vi "cRioMain.vi"() -> ()   [LabVIEW 2020]
uses:
  <vilib>/NIScanEngine/faults/Fault.ctl
  Status_cRio.ctl
  Statusword_status.ctl
  ElementDTD.lvlib
panel:
  out "Magnet":bool
  out "Solenoid":bool
  out "Inputs-velocity_actual_value_carrier":i32
  out "Inputs-position_actual_value 2":i32
  out "Inputs-position_actual_value":i32
  out "Verbindung":bool
  out "Ready":bool
  out "TargetReachedY":bool
  out "StatusY":T1
  out "state change":bool
  out "TargetReachedZ":bool
  out "MotorFault":bool
  out "StatusZ":T1
  in  "turnOffM":bool=TRUE
  in  "halt":bool=TRUE
  out "status":T2=enum."1_start_up"
  out "Turn Off":bool
  out "ZielTisch":dbl
  out "Zielhöhe":dbl
  out "fault list":T3[](array[typedef]) caption="Fehlerliste" {"level" items=["Geringfügiger Fehler", "Schwerer Fehler", "Nicht behebbarer Fehler"]}
  out "pcError":bool
  out "Repair":bool
  out "Start":bool
  in  "Stopp":bool
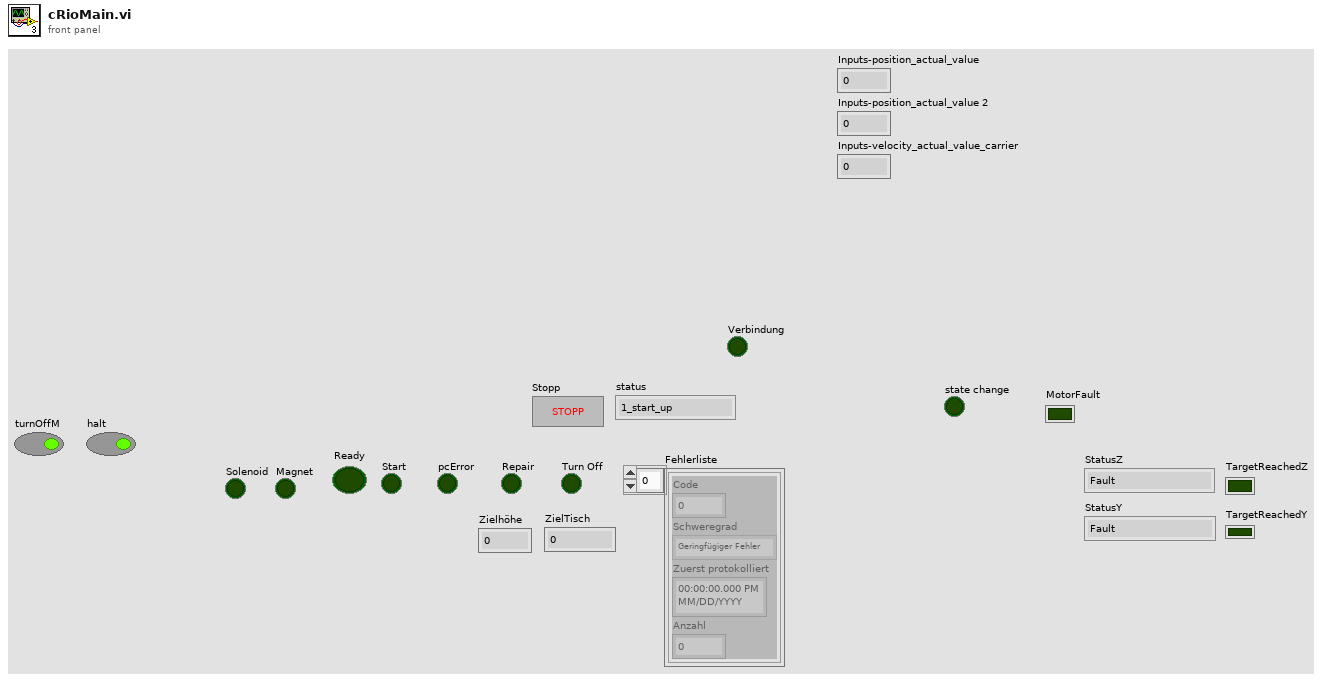
[diagram p1: front panel]
types:
  T1 = typedef "ElementDTD.lvlib/Statusword_status.ctl" = enum16{"Fault", "NOT_READY_TO_SWITCH_ON", "SWITCH_ON_DISABLED", "READY_TO_SWITCH_ON", "SWITCHED_ON", "OPERATION_ENABLE", "QUICK_STOP_ACTIVE"}
  T2 = typedef "ElementDTD.lvlib/Status_cRio.ctl" = enum16{"0_Error", "1_start_up", "4_moving_to_position", "5_measure", "6_DataExport", "7_turnOff"}
  T3 = typedef "Fault.ctl" = cluster{"code":i32, "level":i32, "first reported time":timestamp, "number reported":u32}
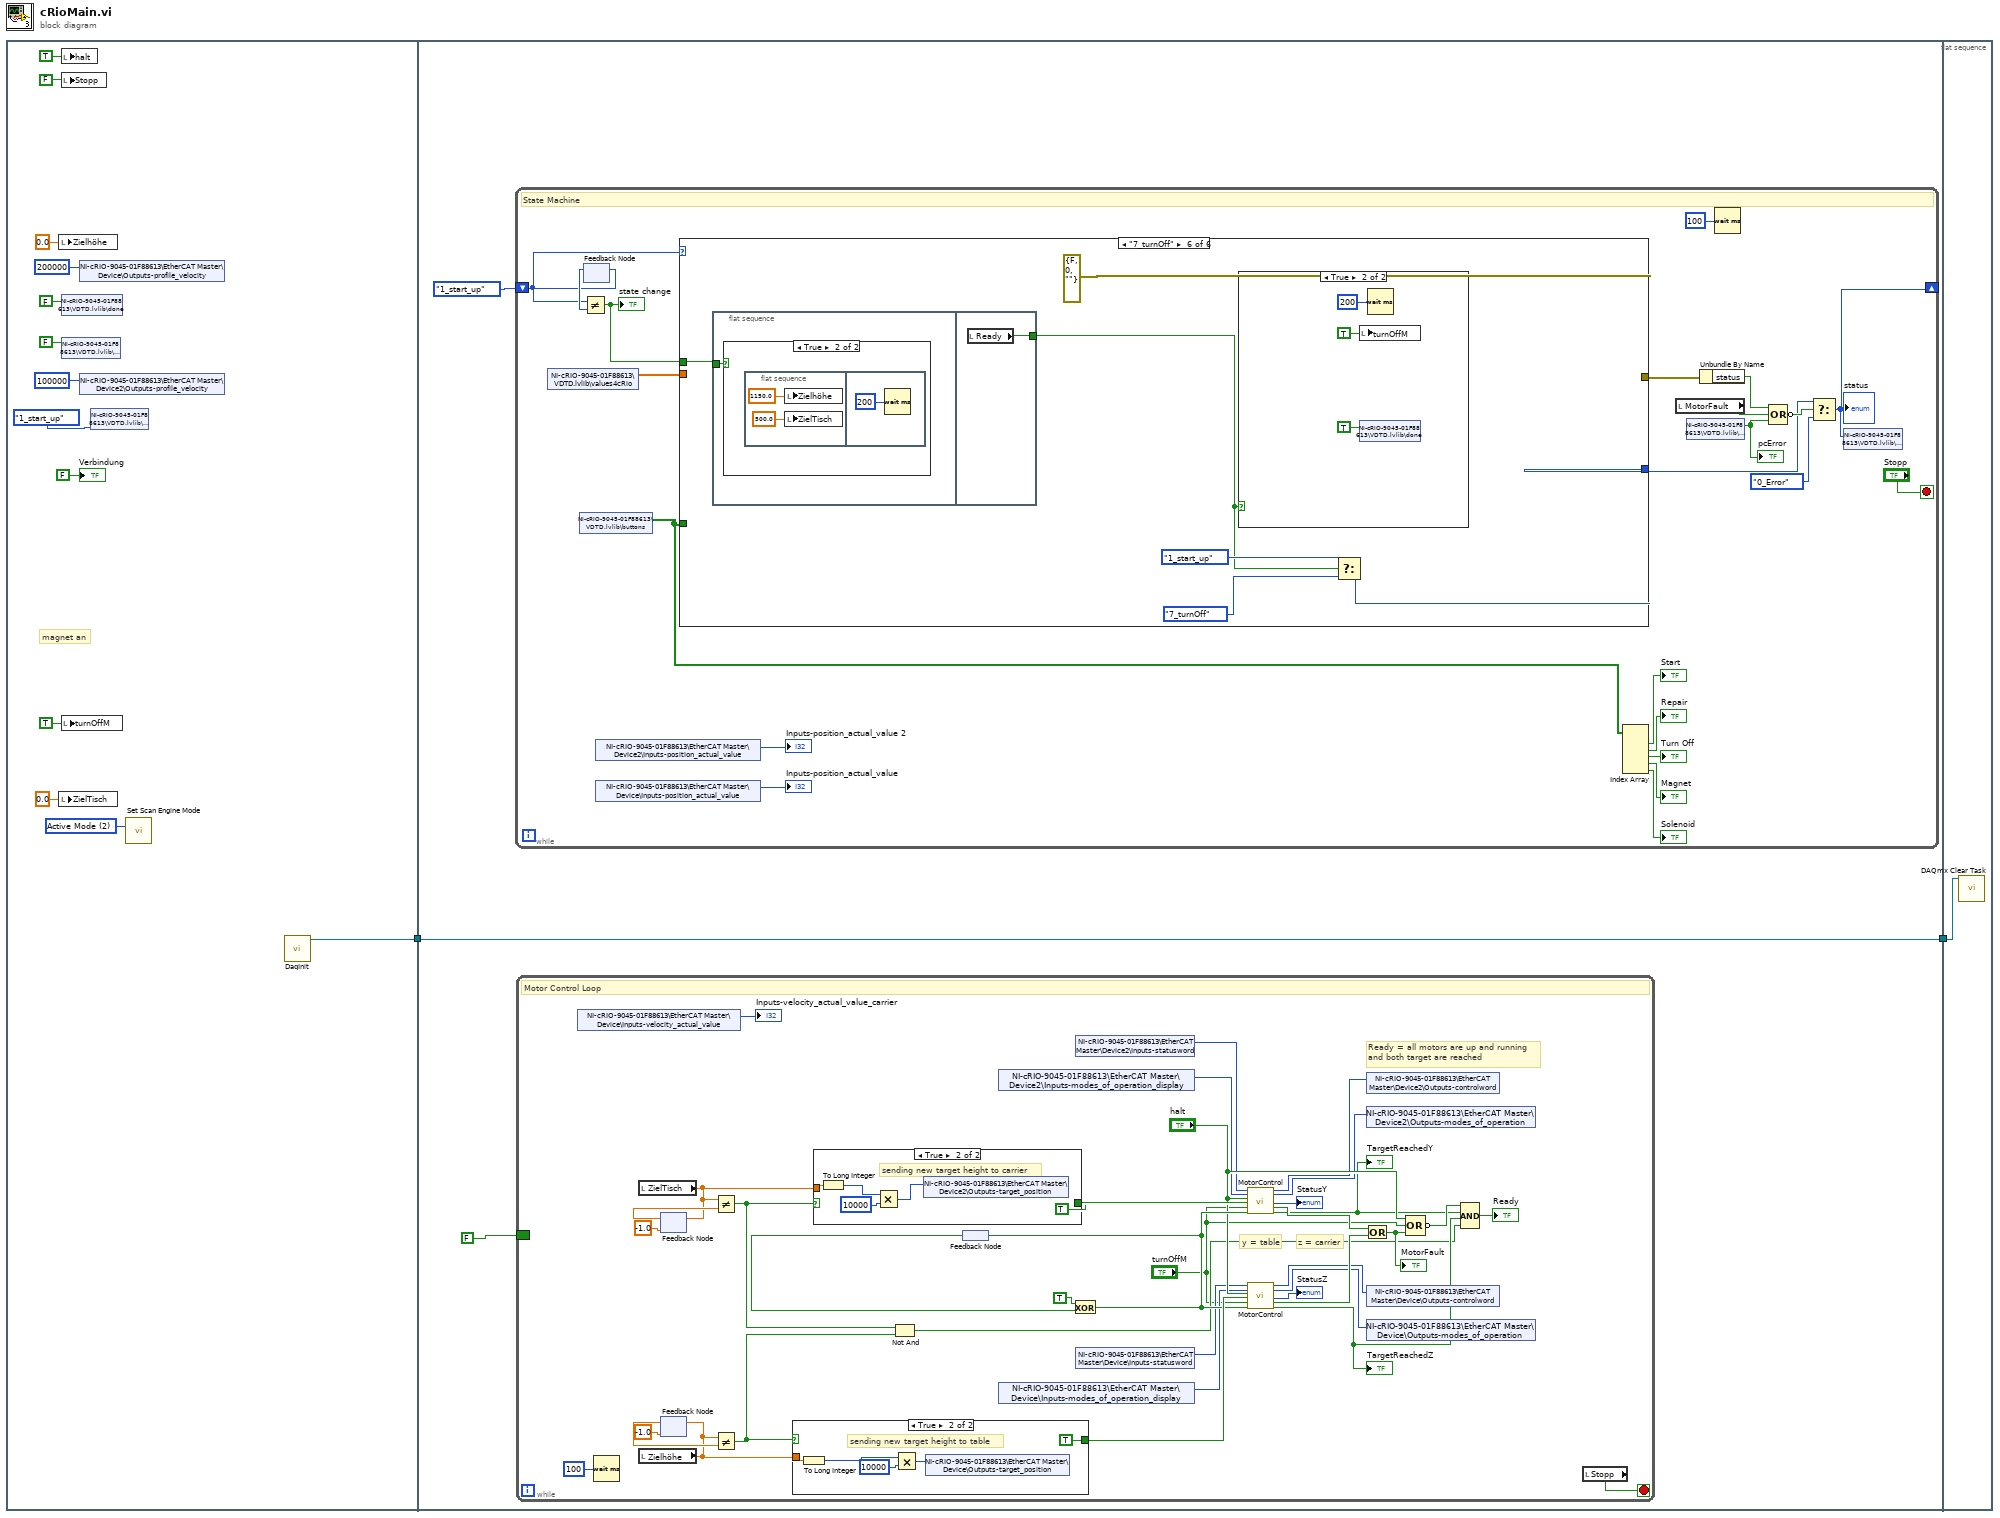
[diagram p0: block diagram]
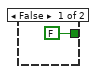
[diagram p2: hidden frame]
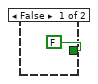
[diagram p3: hidden frame]
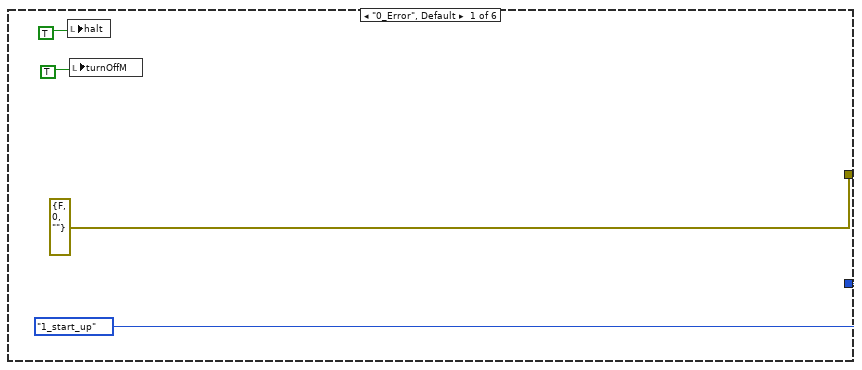
[diagram p4: hidden frame]
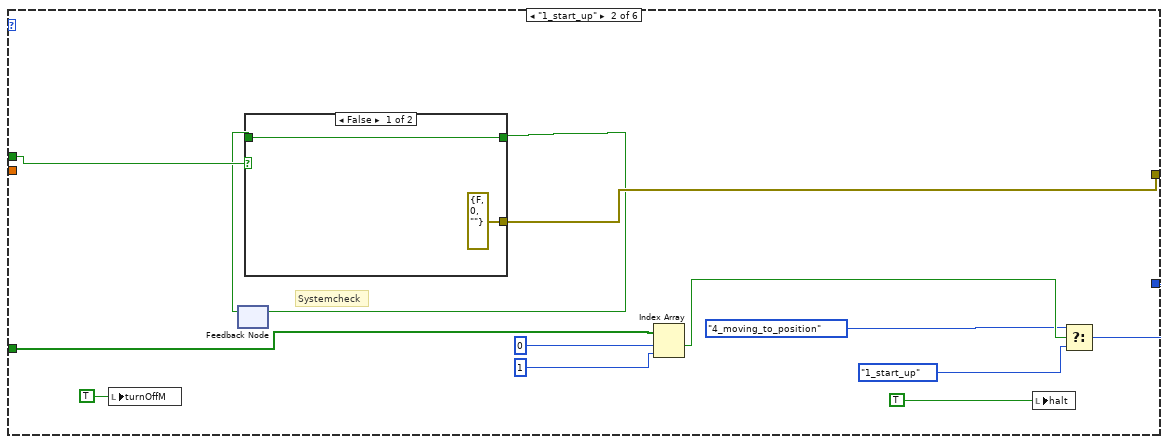
[diagram p5: hidden frame]
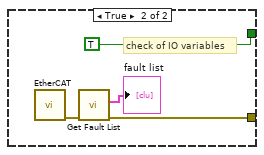
[diagram p6: hidden frame]
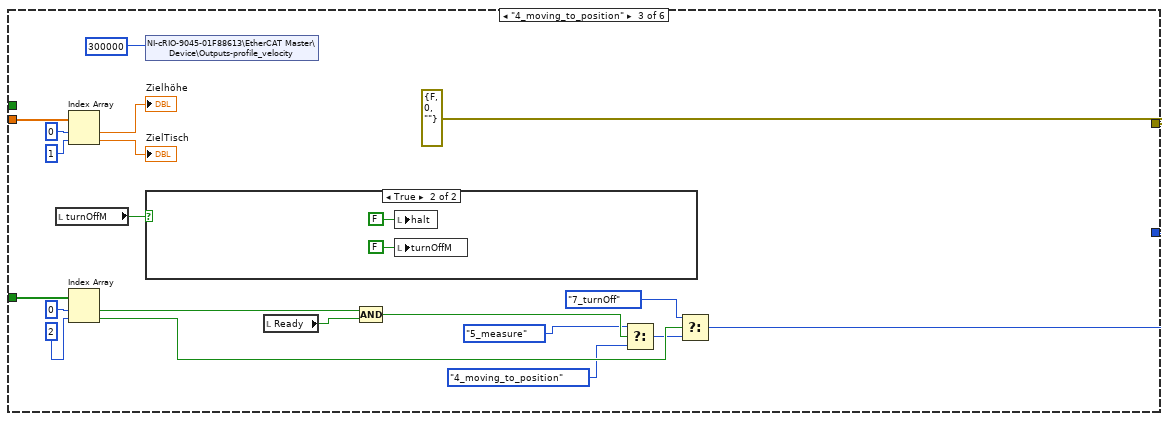
[diagram p7: hidden frame]
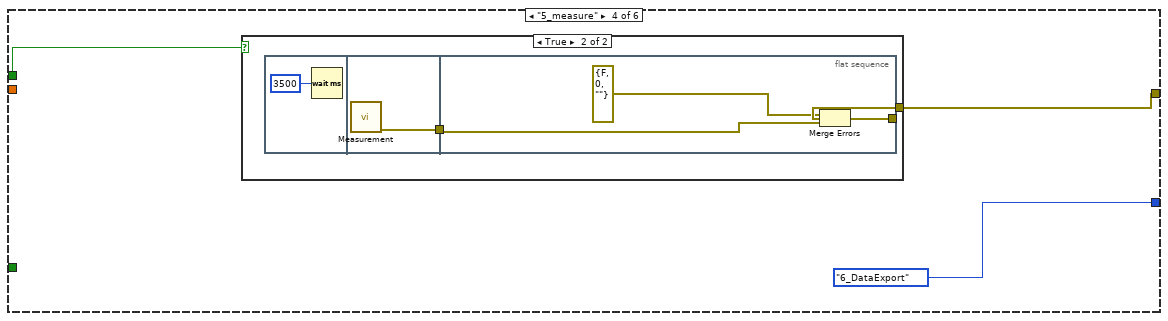
[diagram p9: hidden frame]
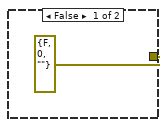
[diagram p10: hidden frame]
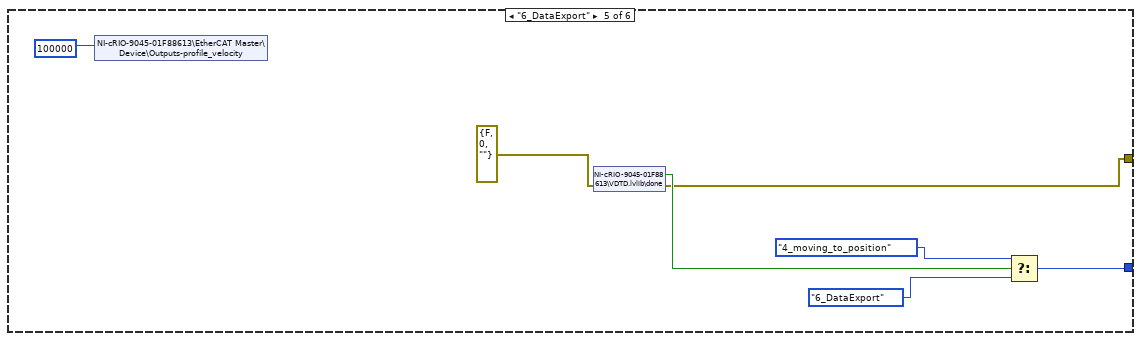
[diagram p11: hidden frame]
diagram:
  n1 = flat-sequence {
    tunnel: [w3] -> w2
    tunnel: w2 -> [w16]
    tunnel: [w16] -> w1
    tunnel: w1 -> [w166]
    frame #0 {
      w6 = 2 items=["Configuration Mode"=1, "Active Mode"=2] ("mode (Active Mode)")
      # "magnet an"
      n2 = local write "Zielhöhe"(0.0 ("Zielhöhe")) -> ()
      n3 = local write "ZielTisch"(0.0 ("ZielTisch")) -> ()
      n4 = local write "halt"(TRUE ("halt")) -> ()
      n5 = local write "Stopp"(FALSE ("Stopp")) -> ()
      n6 = shared-variable "NI-cRIO-9045-01F88613\\VDTD.lvlib\\done"(FALSE ("Done")) -> ()  [unwired: 1 in, 1 out]
      n7 = shared-variable "NI-cRIO-9045-01F88613\\VDTD.lvlib\\error"(FALSE ("Error")) -> ()  [unwired: 1 in, 1 out]
      n8 = local write "turnOffM"(TRUE ("Turn Off")) -> ()
      n9 = shared-variable "NI-cRIO-9045-01F88613\\EtherCAT Master\\Device\\Outputs-profile_velocity"(u32 200000 ("Outputs-profile_velocity")) -> ()  [unwired: 1 in, 1 out]
      n10 = shared-variable "NI-cRIO-9045-01F88613\\EtherCAT Master\\Device2\\Outputs-profile_velocity"(u32 100000 ("Outputs-profile_velocity")) -> ()  [unwired: 1 in, 1 out]
      n11 = shared-variable "NI-cRIO-9045-01F88613\\VDTD.lvlib\\state"(Status_cRio."1_start_up" ("state")) -> ()  [unwired: 1 in, 1 out]
      n12 = call <vilib>:"Set Scan Engine Mode.vi"("mode (Active Mode)"=w6) -> ()  [unwired: 14 in, 1 out]
      n13 = call "DaqInit.vi"() -> ("Refnum out"=w3:refnum<k21>)  [unwired: 10 in, 1 out]
      "Verbindung" <- FALSE ("Verbindung")
    }
    frame #1 {
      n14 = while {
        shift-right: [w73] -> _
        shift-left: Status_cRio."1_start_up" -> [w77]
        stop <- "Stopp" stop-if-true
        # "State Machine"
        n15 = shared-variable "NI-cRIO-9045-01F88613\\VDTD.lvlib\\values4cRio"() -> (w68:dbl[])  [unwired: 1 in, 1 out]
        n16 = shared-variable "NI-cRIO-9045-01F88613\\VDTD.lvlib\\buttons"() -> (w71:bool[])  [unwired: 1 in, 1 out]
        n17 = feedback-in #1(w77) -> ()
        n18 = feedback #1() -> (w80:T2)  [unwired: 1 in]
        n19 = Not Equal?(x=w77, y=w80) -> (x != y?=w72:bool)
        "state change" <- w72
        n20 = shared-variable "NI-cRIO-9045-01F88613\\EtherCAT Master\\Device2\\Inputs-position_actual_value"() -> (→"Inputs-position_actual_value 2":i32)  [unwired: 1 in, 1 out]
        n21 = shared-variable "NI-cRIO-9045-01F88613\\EtherCAT Master\\Device\\Inputs-position_actual_value"() -> (→"Inputs-position_actual_value":i32)  [unwired: 1 in, 1 out]
        n22 = case shown="\"7_turnOff\"" w77 {
          tunnel: [errorcluster {"status"=FALSE, "code"=0, "source"=""} ("error IO") w96 errorcluster {"status"=FALSE, "code"=0, "source"=""} ("error IO") w136 w146 errorcluster {"status"=FALSE, "code"=0, "source"=""} ("error IO")] -> w85
          tunnel: [Status_cRio."1_start_up" w104 w129 Status_cRio."6_DataExport" w145 w154] -> w76
          tunnel: w72 -> [_ w97 _ w135 _ w152]
          tunnel: w71 -> [_ w101 w123 _ _ _]
          tunnel: w68 -> [_ _ w116 _ _ _]
          frame "0_Error", Default {
            n23 = local write "halt"(TRUE ("halt")) -> ()
            n24 = local write "turnOffM"(TRUE ("Turn Off")) -> ()
          }
          frame "1_start_up" {
            # "Systemcheck"
            n25 = local write "turnOffM"(TRUE ("turnOffM")) -> ()
            n26 = feedback #2() -> (w95:bool)  [unwired: 1 in]
            n27 = case shown="False" w97 {
              tunnel: [errorcluster {"status"=FALSE, "code"=0, "source"=""} ("error IO") w110] -> w96
              tunnel: [w106 TRUE ("halt")] -> w94
              tunnel: w95 -> [w106 _]
              frame False {
              }
              frame True {
                # "check of IO variables"
                n28 = call "EtherCAT.vi"() -> ("error IO"=w111:errorcluster)  [unwired: 11 in]
                n29 = call <vilib>:"Get Fault List.vi"("error in (no error)"=w111) -> ("error out"=w110:errorcluster, "fault list"=→"fault list":T3[])  [unwired: 9 in]
              }
            }
            n30 = feedback-in #2(w94) -> ()
            n31 = Index Array(array=w101, index #1=0 ("index"), index #2=1 ("index")) -> (element #1=w100:bool)  [unwired: 1 out]
            n32 = local write "halt"(TRUE ("halt")) -> ()
            n33 = Select(t=Status_cRio."4_moving_to_position", s=w100, f=Status_cRio."1_start_up") -> (s? t:f=w104:T2)
          }
          frame "4_moving_to_position" {
            n34 = local read "turnOffM"() -> (w130:bool)
            n35 = Index Array(array=w116, index #1=0 ("Index"), index #2=1 ("Index")) -> (element #1=→"Zielhöhe":dbl, element #2=→"ZielTisch":dbl)
            n36 = Index Array(array=w123, index #1=0 ("index"), index #2=2 ("index")) -> (element #1=w124:bool, element #2=w121:bool)
            n37 = shared-variable "NI-cRIO-9045-01F88613\\EtherCAT Master\\Device\\Outputs-profile_velocity"(u32 300000 ("Outputs-profile_velocity")) -> ()  [unwired: 1 in, 1 out]
            n38 = case shown="True" w130 {
              frame False {
              }
              frame True {
                n39 = local write "halt"(FALSE ("halt")) -> ()
                n40 = local write "turnOffM"(FALSE ("turnOffM")) -> ()
              }
            }
            n41 = local read "Ready"() -> (w128:bool)
            n42 = Compound Arithmetic op=AND ("Mehrfacharithmetik")(w124, w128) -> (w115:bool)
            n43 = Select(t=Status_cRio."5_measure", s=w115, f=Status_cRio."4_moving_to_position") -> (s? t:f=w112:T2)
            n44 = Select(t=Status_cRio."7_turnOff" ("f"), s=w121, f=w112) -> (s? t:f=w129:T2)
          }
          frame "5_measure" {
            n45 = case shown="True" w135 {
              tunnel: [errorcluster {"status"=FALSE, "code"=0, "source"=""} ("error IO") w139] -> w136
              frame False {
              }
              frame True {
                n46 = flat-sequence {
                  tunnel: [w141] -> w138
                  tunnel: w138 -> [w143]
                  tunnel: [w144] -> w139
                  frame #0 {
                    n47 = Wait (ms)(milliseconds to wait=u32 3500) -> ()  [unwired: 1 out]
                  }
                  frame #1 {
                    n48 = call "Measurement.vi"() -> ("Fehler (Ausgang)"=w141:errorcluster)  [unwired: 11 in]
                  }
                  frame #2 {
                    n49 = Merge Errors(errorcluster {"status"=FALSE, "code"=0, "source"=""} ("error IO"), w143) -> (w144:errorcluster)
                  }
                }
              }
            }
          }
          frame "6_DataExport" {
            n50 = shared-variable "NI-cRIO-9045-01F88613\\EtherCAT Master\\Device\\Outputs-profile_velocity"(u32 100000 ("Outputs-profile_velocity")) -> ()  [unwired: 1 in, 1 out]
            n51 = shared-variable "NI-cRIO-9045-01F88613\\VDTD.lvlib\\done"(error in=errorcluster {"status"=FALSE, "code"=0, "source"=""} ("error IO")) -> (w149:bool, error out=w146:errorcluster)
            n52 = Select(t=Status_cRio."4_moving_to_position", s=w149, f=Status_cRio."6_DataExport") -> (s? t:f=w145:T2)
          }
          frame "7_turnOff" {
            n53 = flat-sequence {
              tunnel: w152 -> [w158]
              tunnel: [w162] -> w153
              frame #0 {
                n54 = case shown="True" w158 {
                  frame False {
                  }
                  frame True {
                    n55 = flat-sequence {
                      frame #0 {
                        n56 = local write "Zielhöhe"(1150.0 ("Zielhöhe")) -> ()
                        n57 = local write "ZielTisch"(500.0 ("ZielTisch")) -> ()
                      }
                      frame #1 {
                        n58 = Wait (ms)(milliseconds to wait=u32 200 ("Zu wartende ms")) -> ()  [unwired: 1 out]
                      }
                    }
                  }
                }
              }
              frame #1 {
                n59 = local read "Ready"() -> (w162:bool)
              }
            }
            n60 = case shown="True" w153 {
              frame False {
              }
              frame True {
                n61 = local write "turnOffM"(TRUE ("turnOffM")) -> ()
                n62 = shared-variable "NI-cRIO-9045-01F88613\\VDTD.lvlib\\done"(TRUE ("Done")) -> ()  [unwired: 1 in, 1 out]
                n63 = Wait (ms)(milliseconds to wait=u32 200) -> ()  [unwired: 1 out]
              }
            }
            n64 = Select(t=Status_cRio."1_start_up", s=w153, f=Status_cRio."7_turnOff") -> (s? t:f=w154:T2)
          }
        }
        n65 = Index Array(array=w71) -> (element #1=→"Start":bool, element #2=→"Repair":bool, element #3=→"Turn Off":bool, element #4=→"Magnet":bool, element #5=→"Solenoid":bool)  [unwired: 5 in]
        n66 = local read "MotorFault"() -> (w84:bool)
        n67 = shared-variable "NI-cRIO-9045-01F88613\\VDTD.lvlib\\error"() -> (w67:bool)  [unwired: 1 in, 1 out]
        "pcError" <- w67
        n68 = Unbundle By Name(w85) -> ("status"=w82:bool)
        n69 = Wait (ms)(milliseconds to wait=u32 100) -> ()  [unwired: 1 out]
        n70 = Compound Arithmetic op=OR(w82, w84, w67) -> (invert w83:bool)
        n71 = Select(t=w76, s=w83, f=Status_cRio."0_Error") -> (s? t:f=w73:T2)
        "status" <- w73
        n72 = shared-variable "NI-cRIO-9045-01F88613\\VDTD.lvlib\\state"(w73) -> ()  [unwired: 1 in, 1 out]
      }
      n73 = while "While-Schleife" {
        border: FALSE -> [_]
        stop <- w51 stop-if-true
        # "Ready = all motors are up and running\nand both target are reached"
        # "y = table"
        # "z = carrier"
        # "Motor Control Loop"
        n74 = shared-variable "NI-cRIO-9045-01F88613\\EtherCAT Master\\Device\\Inputs-velocity_actual_value"() -> (→"Inputs-velocity_actual_value_carrier":i32)  [unwired: 1 in, 1 out]
        n75 = Wait (ms)(milliseconds to wait=u32 100) -> ()  [unwired: 1 out]
        n76 = local read "ZielTisch"() -> (w46:dbl)
        n77 = local read "Zielhöhe"() -> (w50:dbl)
        n78 = feedback #3(-1.0 ("Zielhöhe")) -> (w48:dbl)
        n79 = feedback-in #3(w46) -> ()
        n80 = feedback #4(-1.0 ("Zielhöhe")) -> (w53:dbl)
        n81 = feedback-in #4(w50) -> ()
        n82 = Not Equal?(x=w46, y=w48) -> (x != y?=w24:bool)
        n83 = Not Equal?(x=w50, y=w53) -> (x != y?=w23:bool)
        n84 = case shown="True" w23 {
          tunnel: w50 -> [_ w60]
          tunnel: [FALSE ("new value") TRUE ("new value")] -> w52
          frame False {
          }
          frame True {
            # "sending new target height to table"
            n85 = To Long Integer(number=w60) -> (32bit integer=w59:i32)
            n86 = Multiply(x=w59, y=10000) -> (x*y=w56:i32)
            n87 = shared-variable "NI-cRIO-9045-01F88613\\EtherCAT Master\\Device\\Outputs-target_position"(w56) -> ()  [unwired: 1 in, 1 out]
          }
        }
        n88 = case shown="True" w24 {
          tunnel: w46 -> [_ w64]
          tunnel: [FALSE ("NewValueT") TRUE ("NewValueT")] -> w39
          frame False {
          }
          frame True {
            # "sending new target height to carrier"
            n89 = To Long Integer(number=w64) -> (32bit integer=w66:i32)
            n90 = Multiply(x=w66, y=10000) -> (x*y=w62:i32)
            n91 = shared-variable "NI-cRIO-9045-01F88613\\EtherCAT Master\\Device2\\Outputs-target_position"(w62) -> ()  [unwired: 1 in, 1 out]
          }
        }
        n92 = Not And(1:w23, 2:w24) -> (0:w22:bool)
        n93 = feedback #5() -> (w45:bool)
        n94 = shared-variable "NI-cRIO-9045-01F88613\\EtherCAT Master\\Device2\\Inputs-modes_of_operation_display"() -> (w32:i8)  [unwired: 1 in, 1 out]
        n95 = shared-variable "NI-cRIO-9045-01F88613\\EtherCAT Master\\Device\\Inputs-modes_of_operation_display"() -> (w36:i8)  [unwired: 1 in, 1 out]
        n96 = Exclusive Or(1:w45, 2:TRUE ("x")) -> (0:w43:bool)
        n97 = feedback-in #5(w43) -> ()
        n98 = shared-variable "NI-cRIO-9045-01F88613\\EtherCAT Master\\Device2\\Inputs-statusword"() -> (w31:u16)  [unwired: 1 in, 1 out]
        n99 = shared-variable "NI-cRIO-9045-01F88613\\EtherCAT Master\\Device\\Inputs-statusword"() -> (w35:u16)  [unwired: 1 in, 1 out]
        n100 = call "MotorControl.vi"("Inputs-statusword"=w31, "Inputs-mode_of_operation_display"=w32, "halt"="halt", "new value"=w39, "turn off"="turnOffM", "clock"=w43) -> ("controlword"=w30:u16, "Outputs-mode_of_operation"=w29:i8, "Status"=→"StatusY":T1, "Fault"=w41:bool, "TargetReached"=w26:bool)  [unwired: 9 in]
        "TargetReachedY" <- w26
        n101 = call "MotorControl.vi"("Inputs-statusword"=w35, "Inputs-mode_of_operation_display"=w36, "halt"="halt", "new value"=w52, "turn off"="turnOffM", "clock"=w43) -> ("controlword"=w34:u16, "Outputs-mode_of_operation"=w33:i8, "Status"=→"StatusZ":T1, "Fault"=w42:bool, "TargetReached"=w25:bool)  [unwired: 9 in]
        "TargetReachedZ" <- w25
        n102 = Or(x=w41, y=w42) -> (x .or. y?=w37:bool)
        "MotorFault" <- w37
        n103 = shared-variable "NI-cRIO-9045-01F88613\\EtherCAT Master\\Device2\\Outputs-controlword"(w30) -> ()  [unwired: 1 in, 1 out]
        n104 = shared-variable "NI-cRIO-9045-01F88613\\EtherCAT Master\\Device2\\Outputs-modes_of_operation"(w29) -> ()  [unwired: 1 in, 1 out]
        n105 = shared-variable "NI-cRIO-9045-01F88613\\EtherCAT Master\\Device\\Outputs-controlword"(w34) -> ()  [unwired: 1 in, 1 out]
        n106 = shared-variable "NI-cRIO-9045-01F88613\\EtherCAT Master\\Device\\Outputs-modes_of_operation"(w33) -> ()  [unwired: 1 in, 1 out]
        n107 = Compound Arithmetic op=OR ("Mehrfacharithmetik")("halt", "turnOffM", w37) -> (invert w27:bool)
        n108 = Compound Arithmetic op=AND ("Mehrfacharithmetik")(w27, w26, w25, w22) -> (→"Ready":bool)
        n109 = local read "Stopp"() -> (w51:bool)
      }
    }
    frame #2 {
      n110 = call <vilib>:"DAQmx Clear Task.vi"("task in"=w166) -> ()  [unwired: 14 in, 1 out]
    }
  }
